vi "Created Insert.vi"(9 "Created":refnum<user-event>, 10 "Created Alias":string, 11 "Addresses Strategy in":refnum<class "Addresses Strategy.lvclass">) -> (3 "Addresses Strategy out":refnum<class "Addresses Strategy.lvclass">)   [LabVIEW 2021, in "jettl.lvlib" / "Addresses Strategy.lvlib" / "Addresses Strategy.lvclass"]
uses:
  Addresses Strategy.lvclass
  Msg/Msg.lvclass
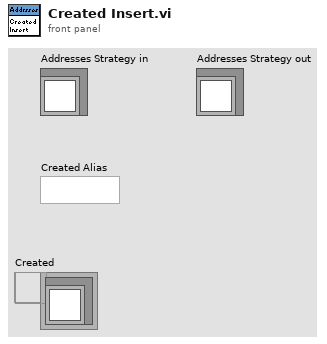
[diagram p1: front panel]
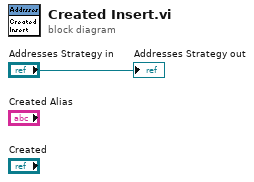
[diagram p0: block diagram]
diagram:
  "Addresses Strategy out" <- "Addresses Strategy in"
